vi "variant to json.vi"(7 "options":T1, 8 "error in (no error)":errorcluster, 11 "Variant":variant) -> (0 "error out":errorcluster, 3 "JSON Value":refnum<class "JSON Value.lvclass">)   [LabVIEW 2016, in "JSON Variant Support.lvclass"]
uses:
  JSON Variant Support.lvclass
  JSON Value/JSON Value.lvclass
  <vilib>/Utility/Data Type/Type Definitions/Data Type.ctl
  JSON Value/New JSON Value/New JSON (Null).vi
  JSON Value/New JSON Value/New JSON (Numeric).vi
  JSON Value/New JSON Value/New JSON (Boolean).vi
  JSON Value/New JSON Value/New JSON (String).vi
  JSON Value/New JSON Value/New JSON (Value[]).vi
  JSON Value/New JSON Value/New JSON ({Value[]}).vi
  <vilib>/Utility/Data Type/NI_Data Type.lvlib
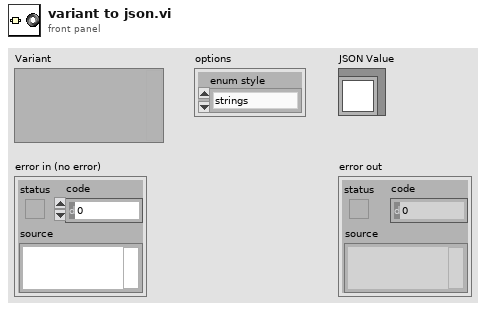
[diagram p1: front panel]
types:
  T1 = cluster{"enum style":enum16{"strings", "numbers", "both"}}
  T2 = typedef "NI_Data Type.lvlib/Data Type.ctl" = enum8{"Invalid Type", "Void", "I8", "I16", "I32", "I64", "U8", "U16", "U32", "U64", "Single Float", "Double Float", "Extended Float", "Single Complex", "Double Complex", "Extended Complex", "Enum U8", "Enum U16", "Enum U32", "Enum U64", "Single Float With Unit", "Double Float With Unit", "Extended Float With Unit", "Single Complex with Unit", "Double Complex with Unit", "Extended Complex with Unit", "Boolean", "String", "Path", "Picture", "Tag", "Array", "Cluster", "Variant", "LV Variant", "Waveform", "Timestamp", "Digital Waveform", "Digital Data", "ExpressData", "Refnum", "External Data", "VI", "Poly VI", "LabVIEW Class Instance", "Fixed Point"}
  T3 = typedef "imagedata.ctl" = cluster{"image type":i32, "image depth":i32, "image":u8[], "mask":u8[], "colors":u32[], "Rectangle":cluster{"left":i16, "top":i16, "right":i16, "bottom":i16}}
  T4 = typedef "LVFixedPointRepRangeTypeDef.ctl" = cluster{"Range Min":dbl, "Range Max":dbl, "Delta":dbl}
  T5 = typedef "LVFixedPointRepBitsTypeDef.ctl" = cluster{"Signed":bool, "Word Length":u32, "Integer Word Length":i32}
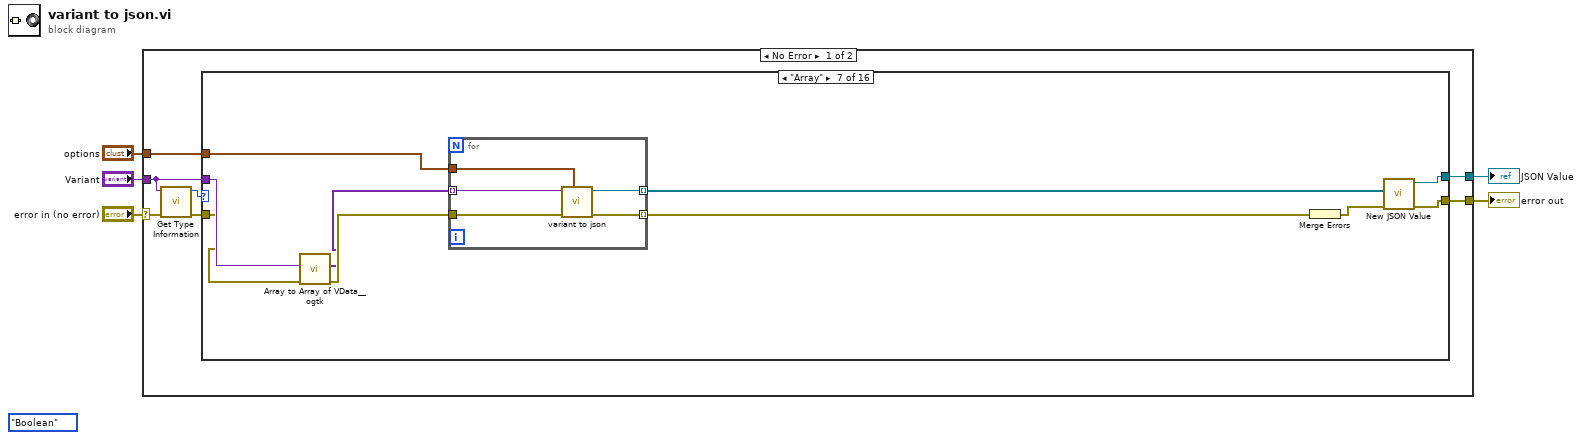
[diagram p0: block diagram]
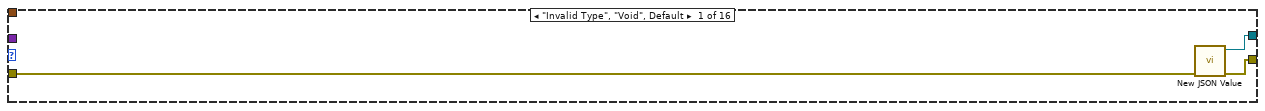
[diagram p2: hidden frame]
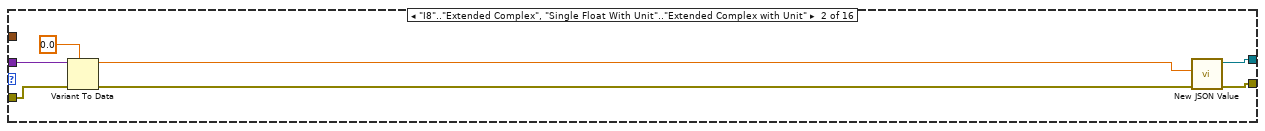
[diagram p3: hidden frame]
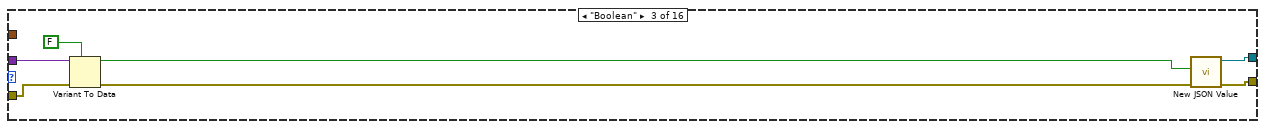
[diagram p4: hidden frame]
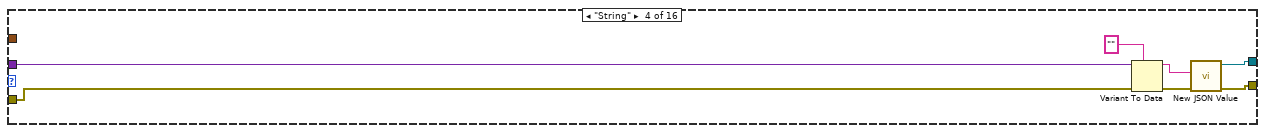
[diagram p5: hidden frame]
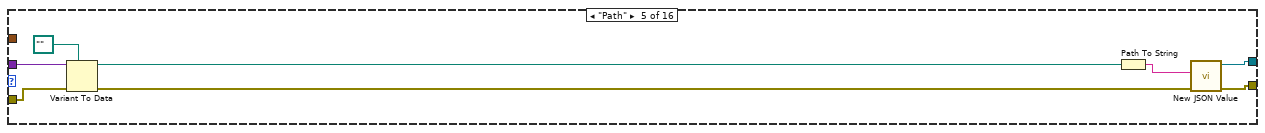
[diagram p6: hidden frame]
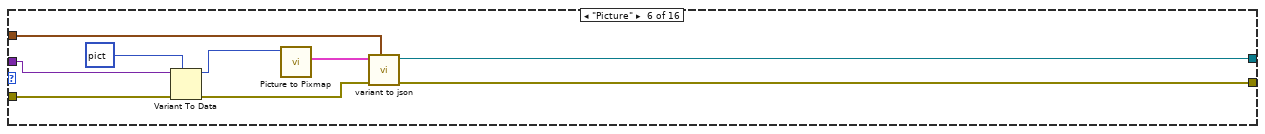
[diagram p7: hidden frame]
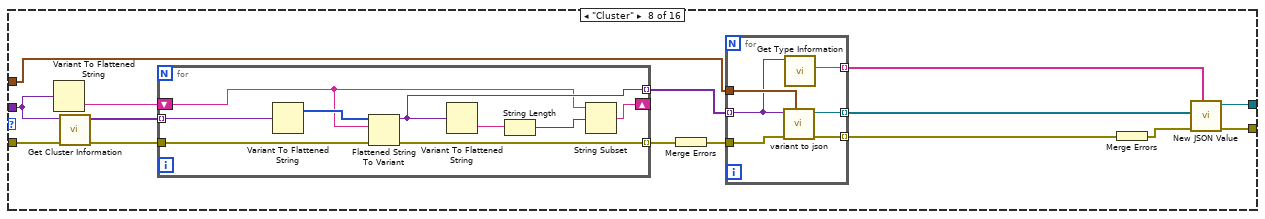
[diagram p8: hidden frame]
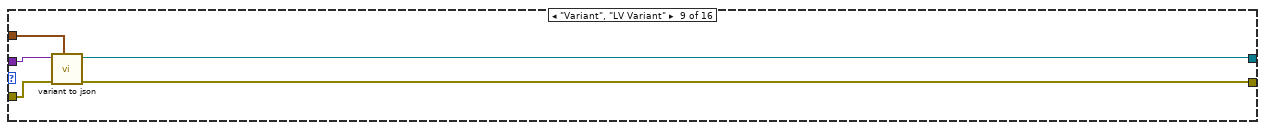
[diagram p9: hidden frame]
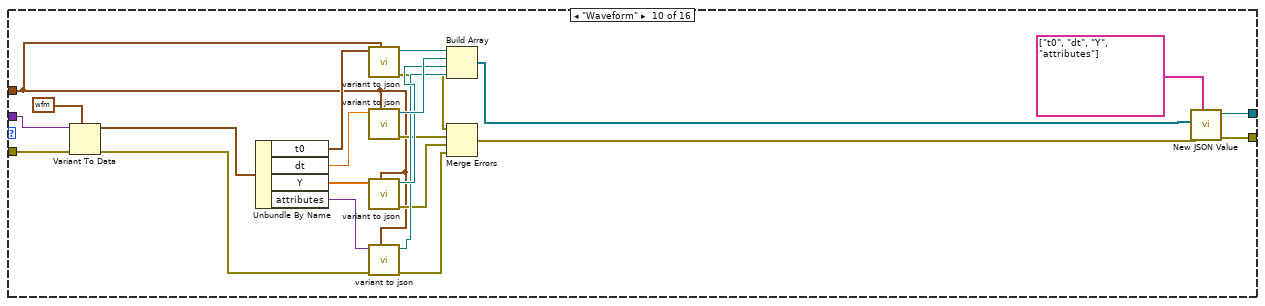
[diagram p10: hidden frame]
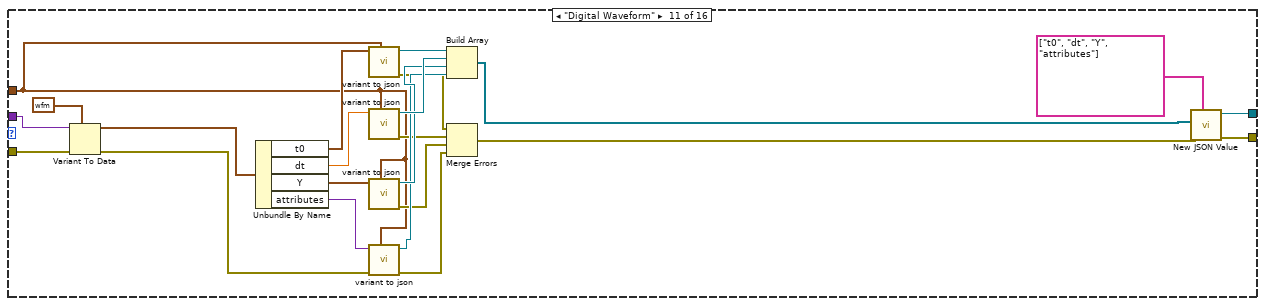
[diagram p11: hidden frame]
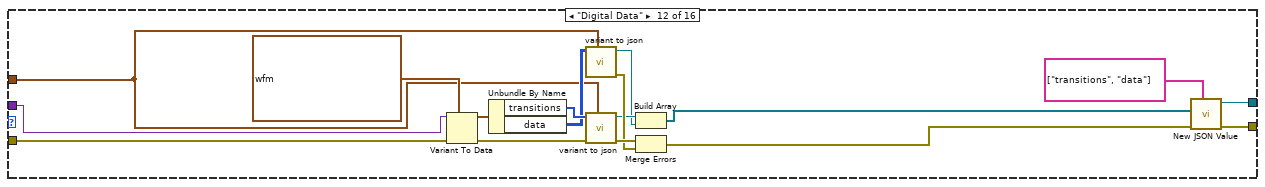
[diagram p12: hidden frame]
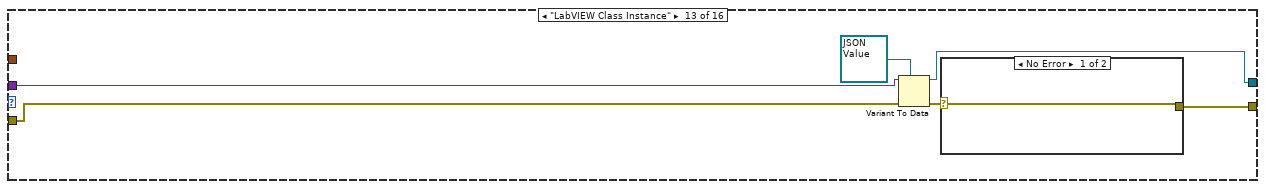
[diagram p13: hidden frame]
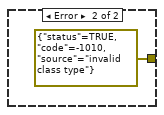
[diagram p14: hidden frame]
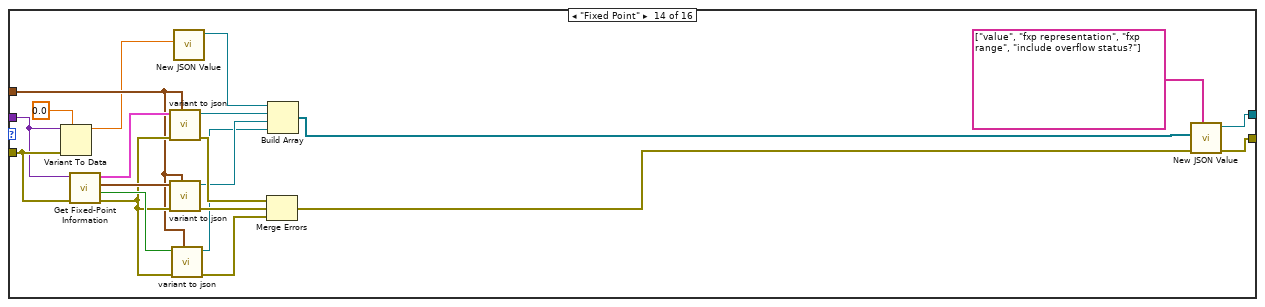
[diagram p15: hidden frame]
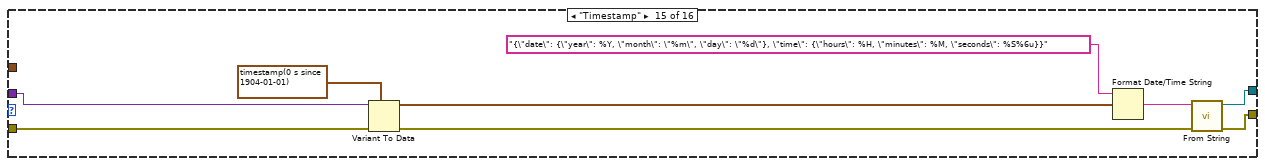
[diagram p16: hidden frame]
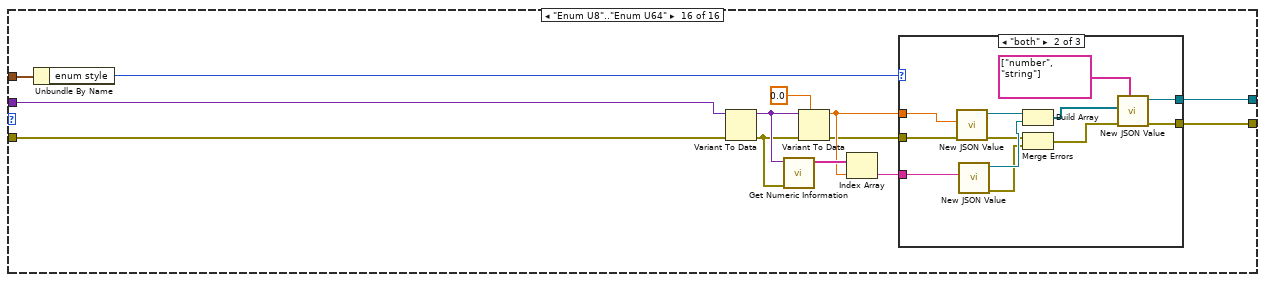
[diagram p17: hidden frame]
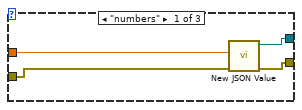
[diagram p18: hidden frame]
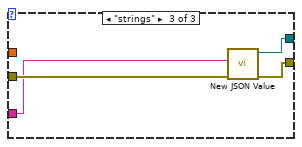
[diagram p19: hidden frame]
diagram:
  (unwired) Data_Type."Boolean" ("Type")
  n1 = case shown="No Error" "error in (no error)" {
    selector: "error in (no error)" -> [w9 w238]
    tunnel: [w8 w238] -> w4
    tunnel: "Variant" -> [w7 _]
    tunnel: [w11 _] -> w2
    tunnel: "options" -> [w6 _]
    frame No Error {
      n2 = call <vilib>:"Get Type Information.vi"("error in (no error)"=w9, "Variant"=w7) -> ("error out"=w10:errorcluster, "Type"=w12:T2)  [unwired: 5 in, 3 out]
      n3 = case shown="\"Digital Data\"" w12 {
        tunnel: [w15 w19 w26 w33 w41 w48 w62 w82 w100 w112 w136 w152 w169 w177 w198 w208] -> w11
        tunnel: w10 -> [w14 w16 w28 w35 w43 w52 w56 w71 w101 w126 w149 w165 w171 w185 w203 w216]
        tunnel: [w13 w18 w25 w32 w40 w46 w61 w81 w103 w111 w135 w153 w167 w176 w197 w207] -> w8
        tunnel: w7 -> [_ w22 w29 w36 w44 w53 w57 w72 w102 w125 w148 w166 w172 w184 w204 w217]
        tunnel: w6 -> [_ _ _ _ _ w45 w58 w70 w99 w104 w128 w159 _ w190 _ w211]
        frame "Invalid Type", "Void", Default {
          n4 = call-poly "New JSON Value.vi"("error in (no error)"=w14) -> ("error out"=w13:errorcluster, "JSON Value out"=w15:refnum<class "JSON Value.lvclass">)  [unwired: 9 in]
        }
        frame "I8".."Extended Complex", "Single Float With Unit".."Extended Complex with Unit" {
          n5 = Variant To Data(error in=w16, type=0.0, Variant=w22) -> (data=w20:dbl, error out=w17:errorcluster)
          n6 = call-poly "New JSON Value.vi"("error in (no error)"=w17, "value"=w20) -> ("error out"=w18:errorcluster, "JSON Value out"=w19:refnum<class "JSON Value.lvclass">)  [unwired: 8 in]
        }
        frame "Boolean" {
          n7 = Variant To Data(error in=w28, type=FALSE, Variant=w29) -> (data=w27:bool, error out=w24:errorcluster)
          n8 = call-poly "New JSON Value.vi"("error in (no error)"=w24, "value"=w27) -> ("error out"=w25:errorcluster, "JSON Value out"=w26:refnum<class "JSON Value.lvclass">)  [unwired: 8 in]
        }
        frame "String" {
          n9 = Variant To Data(error in=w35, type="", Variant=w36) -> (data=w34:string, error out=w31:errorcluster)
          n10 = call-poly "New JSON Value.vi"("error in (no error)"=w31, "value"=w34) -> ("error out"=w32:errorcluster, "JSON Value out"=w33:refnum<class "JSON Value.lvclass">)  [unwired: 8 in]
        }
        frame "Path" {
          n11 = Variant To Data(error in=w43, type=path "", Variant=w44) -> (data=w42:path, error out=w39:errorcluster)
          n12 = Path To String(path=w42) -> (string=w37:string)
          n13 = call-poly "New JSON Value.vi"("error in (no error)"=w39, "value"=w37) -> ("error out"=w40:errorcluster, "JSON Value out"=w41:refnum<class "JSON Value.lvclass">)  [unwired: 8 in]
        }
        frame "Picture" {
          n14 = Variant To Data(error in=w52, type=picture data[5B] ("2D Picture"), Variant=w53) -> (data=w50:picture, error out=w47:errorcluster)
          n15 = call <vilib>:"Picture to Pixmap.vi"("picture"=w50) -> ("image data"=w49:T3)  [unwired: 9 in, 1 out]
          n16 = call "variant to json.vi"("options"=w45, "error in (no error)"=w47, "Variant"=w49) -> ("error out"=w46:errorcluster, "JSON Value"=w48:refnum<class "JSON Value.lvclass">)  [unwired: 7 in]
        }
        frame "Array" {
          n17 = call <userlib>:"Array to Array of VData__ogtk.vi"("error in (no error)"=w56, "MultiD Array"=w57) -> ("error out"=w55:errorcluster, "1D Array of Variants"=w54:variant[])  [unwired: 8 in]
          n18 = for {
            tunnel: w54 -> [w68] mode=indexing
            tunnel: [w67] -> w63 mode=indexing
            tunnel: [w66] -> w60 mode=indexing
            tunnel: w55 -> [w65]
            tunnel: w58 -> [w64]
            n19 = call "variant to json.vi"("options"=w64, "error in (no error)"=w65, "Variant"=w68) -> ("error out"=w66:errorcluster, "JSON Value"=w67:refnum<class "JSON Value.lvclass">)  [unwired: 7 in]
          }
          n20 = Merge Errors(w60) -> (w59:errorcluster)
          n21 = call-poly "New JSON Value.vi"("error in (no error)"=w59, "JSON Datatypes"=w63) -> ("error out"=w61:errorcluster, "JSON Value out"=w62:refnum<class "JSON Value.lvclass">)  [unwired: 8 in]
        }
        frame "Cluster" {
          n22 = Variant To Flattened String(Variant=w72) -> (data string=w78:string)  [unwired: 1 out]
          n23 = call <vilib>:"Get Cluster Information.vi"("error in (no error)"=w71, "Variant"=w72) -> ("error out"=w76:errorcluster, "Cluster Elements"=w77:variant[])  [unwired: 8 in]
          n24 = for {
            tunnel: w77 -> [w92] mode=indexing
            tunnel: [w90] -> w74 mode=indexing
            shift-right: [w86] -> _
            shift-left: w78 -> [w89]
            tunnel: w76 -> [w85]
            tunnel: [w84] -> w75 mode=indexing
            n25 = Variant To Flattened String(Variant=w92) -> (1:w91:i16[])  [unwired: 1 out]
            n26 = Flattened String To Variant(4:w85, 6:w89, 7:w91) -> (0:w84:errorcluster, 3:w90:variant)
            n27 = Variant To Flattened String(Variant=w90) -> (data string=w88:string)  [unwired: 1 out]
            n28 = String Length(string=w88) -> (length=w87:i32)
            n29 = String Subset(string=w89, offset (0)=w87) -> (substring=w86:string)  [unwired: 1 in]
          }
          n30 = Merge Errors(w75) -> (w73:errorcluster)
          n31 = for {
            tunnel: [w98] -> w83 mode=indexing
            tunnel: [w97] -> w80 mode=indexing
            tunnel: w74 -> [w94] mode=indexing
            tunnel: w73 -> [w96]
            tunnel: w70 -> [w95]
            tunnel: [w93] -> w69 mode=indexing
            n32 = call "variant to json.vi"("options"=w95, "error in (no error)"=w96, "Variant"=w94) -> ("error out"=w97:errorcluster, "JSON Value"=w98:refnum<class "JSON Value.lvclass">)  [unwired: 7 in]
            n33 = call <vilib>:"Get Type Information.vi"("Variant"=w94) -> ("Name"=w93:string)  [unwired: 6 in, 4 out]
          }
          n34 = Merge Errors(w80) -> (w79:errorcluster)
          n35 = call-poly "New JSON Value.vi"("keys"=w69, "error in (no error)"=w79, "values"=w83) -> ("error out"=w81:errorcluster, "JSON Value out"=w82:refnum<class "JSON Value.lvclass">)  [unwired: 7 in]
        }
        frame "Variant", "LV Variant" {
          n36 = call "variant to json.vi"("options"=w99, "error in (no error)"=w101, "Variant"=w102) -> ("error out"=w103:errorcluster, "JSON Value"=w100:refnum<class "JSON Value.lvclass">)  [unwired: 7 in]
        }
        frame "Waveform" {
          n37 = Variant To Data(error in=w126, type=waveform(dbl) {"t0"=timestamp(0 s since 1904-01-01), "dt"=1.0, "Y"=[]} ("Waveform"), Variant=w125) -> (data=w123:waveform(dbl), error out=w105:errorcluster)
          n38 = Unbundle By Name(w123) -> ("t0"=w121:timestamp, "dt"=w120:dbl, "Y"=w119:dbl[], "attributes"=w122:variant)
          n39 = call "variant to json.vi"("options"=w104, "Variant"=w121) -> ("error out"=w110:errorcluster, "JSON Value"=w118:refnum<class "JSON Value.lvclass">)  [unwired: 8 in]
          n40 = call "variant to json.vi"("options"=w104, "Variant"=w120) -> ("error out"=w109:errorcluster, "JSON Value"=w117:refnum<class "JSON Value.lvclass">)  [unwired: 8 in]
          n41 = call "variant to json.vi"("options"=w104, "Variant"=w119) -> ("error out"=w108:errorcluster, "JSON Value"=w116:refnum<class "JSON Value.lvclass">)  [unwired: 8 in]
          n42 = call "variant to json.vi"("options"=w104, "error in (no error)"=w105, "Variant"=w122) -> ("error out"=w107:errorcluster, "JSON Value"=w115:refnum<class "JSON Value.lvclass">)  [unwired: 7 in]
          n43 = Build Array(w118, w117, w116, w115) -> (w114:refnum<class "JSON Value.lvclass">[])
          n44 = Merge Errors(w110, w109, w108, w107) -> (w106:errorcluster)
          n45 = call-poly "New JSON Value.vi"("keys"=string[] ["t0", "dt", "Y", "attributes"], "error in (no error)"=w106, "values"=w114) -> ("error out"=w111:errorcluster, "JSON Value out"=w112:refnum<class "JSON Value.lvclass">)  [unwired: 7 in]
        }
        frame "Digital Waveform" {
          n46 = Variant To Data(error in=w149, type=digitalwaveform {"t0"=timestamp(0 s since 1904-01-01), "dt"=0.0, "Y"={"transitions"=[], "data"=[]}} ("waveform"), Variant=w148) -> (data=w147:digitalwaveform, error out=w129:errorcluster)
          n47 = Unbundle By Name(w147) -> ("t0"=w145:timestamp, "dt"=w144:dbl, "Y"=w143:digitaldata, "attributes"=w146:variant)
          n48 = call "variant to json.vi"("options"=w128, "Variant"=w145) -> ("error out"=w134:errorcluster, "JSON Value"=w142:refnum<class "JSON Value.lvclass">)  [unwired: 8 in]
          n49 = call "variant to json.vi"("options"=w128, "Variant"=w144) -> ("error out"=w133:errorcluster, "JSON Value"=w141:refnum<class "JSON Value.lvclass">)  [unwired: 8 in]
          n50 = call "variant to json.vi"("options"=w128, "Variant"=w143) -> ("error out"=w132:errorcluster, "JSON Value"=w140:refnum<class "JSON Value.lvclass">)  [unwired: 8 in]
          n51 = call "variant to json.vi"("options"=w128, "error in (no error)"=w129, "Variant"=w146) -> ("error out"=w131:errorcluster, "JSON Value"=w139:refnum<class "JSON Value.lvclass">)  [unwired: 7 in]
          n52 = Build Array(w142, w141, w140, w139) -> (w138:refnum<class "JSON Value.lvclass">[])
          n53 = Merge Errors(w134, w133, w132, w131) -> (w130:errorcluster)
          n54 = call-poly "New JSON Value.vi"("keys"=string[] ["t0", "dt", "Y", "attributes"], "error in (no error)"=w130, "values"=w138) -> ("error out"=w135:errorcluster, "JSON Value out"=w136:refnum<class "JSON Value.lvclass">)  [unwired: 7 in]
        }
        frame "Digital Data" {
          n55 = Variant To Data(error in=w165, type=digitaldata {"transitions"=[], "data"=[]} ("waveform"), Variant=w166) -> (data=w163:digitaldata, error out=w160:errorcluster)
          n56 = Unbundle By Name(w163) -> ("transitions"=w162:u32[], "data"=w161:u8[][])
          n57 = call "variant to json.vi"("options"=w159, "Variant"=w161) -> ("error out"=w157:errorcluster, "JSON Value"=w155:refnum<class "JSON Value.lvclass">)  [unwired: 8 in]
          n58 = call "variant to json.vi"("options"=w159, "error in (no error)"=w160, "Variant"=w162) -> ("error out"=w158:errorcluster, "JSON Value"=w156:refnum<class "JSON Value.lvclass">)  [unwired: 7 in]
          n59 = Build Array(w156, w155) -> (w151:refnum<class "JSON Value.lvclass">[])
          n60 = Merge Errors(w158, w157) -> (w154:errorcluster)
          n61 = call-poly "New JSON Value.vi"("keys"=string[] ["transitions", "data"], "error in (no error)"=w154, "values"=w151) -> ("error out"=w153:errorcluster, "JSON Value out"=w152:refnum<class "JSON Value.lvclass">)  [unwired: 7 in]
        }
        frame "LabVIEW Class Instance" {
          n62 = Variant To Data(error in=w171, type=refnum<class "JSON Value.lvclass"> refnum ("JSON Value"), Variant=w172) -> (data=w169:refnum<class "JSON Value.lvclass">, error out=w168:errorcluster)
          n63 = case shown="No Error" w168 {
            selector: w168 -> [w173 _]
            tunnel: [w173 errorcluster {"status"=TRUE, "code"=-1010, "source"="invalid class type"} ("error IO")] -> w167
            frame No Error {
            }
            frame Error {
            }
          }
        }
        frame "Fixed Point" {
          n64 = Variant To Data(error in=w185, type=0.0, Variant=w184) -> (data=w183:dbl)  [unwired: 1 out]
          n65 = call <vilib>:"Get Fixed-Point Information.vi"("error in (no error)"=w185, "Variant"=w184) -> ("error out"=w191:errorcluster, "Include Overflow Status?"=w192:bool, "FXP Range"=w193:T4, "FXP Representation"=w194:T5)  [unwired: 6 in]
          n66 = call "variant to json.vi"("options"=w190, "error in (no error)"=w191, "Variant"=w194) -> ("error out"=w189:errorcluster, "JSON Value"=w181:refnum<class "JSON Value.lvclass">)  [unwired: 7 in]
          n67 = call "variant to json.vi"("options"=w190, "error in (no error)"=w191, "Variant"=w193) -> ("error out"=w188:errorcluster, "JSON Value"=w180:refnum<class "JSON Value.lvclass">)  [unwired: 7 in]
          n68 = call "variant to json.vi"("options"=w190, "error in (no error)"=w191, "Variant"=w192) -> ("error out"=w187:errorcluster, "JSON Value"=w179:refnum<class "JSON Value.lvclass">)  [unwired: 7 in]
          n69 = call-poly "New JSON Value.vi"("value"=w183) -> ("JSON Value out"=w182:refnum<class "JSON Value.lvclass">)  [unwired: 9 in, 1 out]
          n70 = Merge Errors(w189, w188, w187) -> (w186:errorcluster)
          n71 = Build Array(w182, w181, w180, w179) -> (w178:refnum<class "JSON Value.lvclass">[])
          n72 = call-poly "New JSON Value.vi"("keys"=string[] ["value", "fxp representation", "fxp range", "include overflow status?"], "error in (no error)"=w186, "values"=w178) -> ("error out"=w176:errorcluster, "JSON Value out"=w177:refnum<class "JSON Value.lvclass">)  [unwired: 7 in]
        }
        frame "Timestamp" {
          n73 = Variant To Data(error in=w203, type=timestamp(0 s since 1904-01-01), Variant=w204) -> (data=w200:timestamp, error out=w199:errorcluster)
          n74 = Format Date/Time String(time format string (%c)="{\"date\": {\"year\": %Y, \"month\": \"%m\", \"day\": \"%d\"}, \"time\": {\"hours\": %H, \"minutes\": %M, \"seconds\": %S%6u}}", seconds (now)=w200) -> (date/time string=w196:string)  [unwired: 1 in]
          n75 = call "From String.vi"("error in (no error)"=w199, "JSON String"=w196) -> ("error out"=w197:errorcluster, "JSON Value out"=w198:refnum<class "JSON Value.lvclass">)  [unwired: 8 in]
        }
        frame "Enum U8".."Enum U64" {
          n76 = Unbundle By Name(w211) -> ("enum style"=w210:enum16{"strings", "numbers", "both"})
          n77 = Variant To Data(error in=w216, Variant=w217) -> (data=w215:variant, error out=w213:errorcluster)  [unwired: 1 in]
          n78 = call <vilib>:"Get Numeric Information.vi"("error in (no error)"=w213, "Variant"=w215) -> ("Enum Names"=w212:string[])  [unwired: 6 in, 3 out]
          n79 = Variant To Data(error in=w213, type=0.0, Variant=w215) -> (data=w209:dbl, error out=w206:errorcluster)
          n80 = Index Array(array=w212, index=w209) -> (element=w205:string)
          n81 = case shown="\"both\"" w210 {
            tunnel: w209 -> [w221 w233 _]
            tunnel: [w220 w226 w237] -> w208
            tunnel: [w219 w222 w236] -> w207
            tunnel: w206 -> [w218 w232 w235]
            tunnel: w205 -> [_ w231 w234]
            frame "numbers" {
              n82 = call-poly "New JSON Value.vi"("error in (no error)"=w218, "value"=w221) -> ("error out"=w219:errorcluster, "JSON Value out"=w220:refnum<class "JSON Value.lvclass">)  [unwired: 8 in]
            }
            frame "both" {
              n83 = call-poly "New JSON Value.vi"("error in (no error)"=w232, "value"=w233) -> ("error out"=w225:errorcluster, "JSON Value out"=w230:refnum<class "JSON Value.lvclass">)  [unwired: 8 in]
              n84 = call-poly "New JSON Value.vi"("value"=w231) -> ("error out"=w224:errorcluster, "JSON Value out"=w229:refnum<class "JSON Value.lvclass">)  [unwired: 9 in]
              n85 = Build Array(w230, w229) -> (w228:refnum<class "JSON Value.lvclass">[])
              n86 = Merge Errors(w225, w224) -> (w223:errorcluster)
              n87 = call-poly "New JSON Value.vi"("keys"=string[] ["number", "string"], "error in (no error)"=w223, "values"=w228) -> ("error out"=w222:errorcluster, "JSON Value out"=w226:refnum<class "JSON Value.lvclass">)  [unwired: 7 in]
            }
            frame "strings" {
              n88 = call-poly "New JSON Value.vi"("error in (no error)"=w235, "value"=w234) -> ("error out"=w236:errorcluster, "JSON Value out"=w237:refnum<class "JSON Value.lvclass">)  [unwired: 8 in]
            }
          }
        }
      }
    }
    frame Error {
    }
  }
  "error out" <- w4
  "JSON Value" <- w2
